vi "arm_sine.vi"(9 "Peak Amp":dbl=1e-05 format="%#_6e", 10 "Freq":dbl=71.34 format="%#_6e", 11 "Keithley":refnum<visa-resource-name>="GPIB1::22::INSTR") -> ()   [LabVIEW 2019]
uses:
  SineGlobals.vi
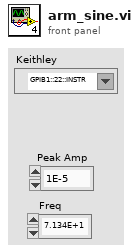
[diagram p1: front panel]
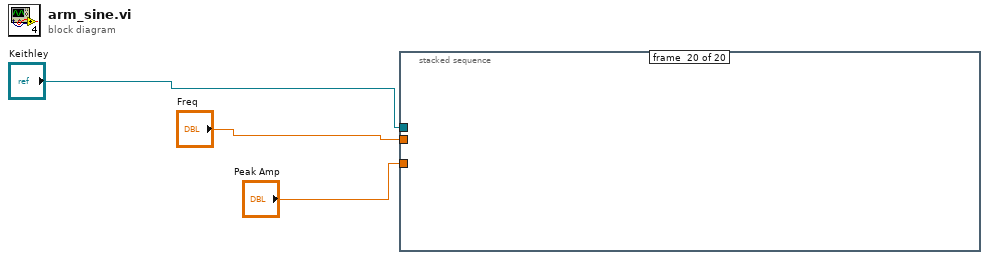
[diagram p0: block diagram]
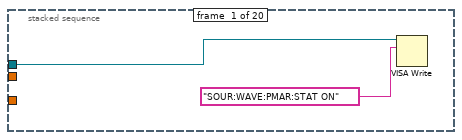
[diagram p2: hidden frame]
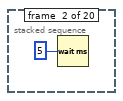
[diagram p3: hidden frame]
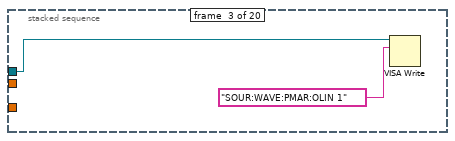
[diagram p4: hidden frame]
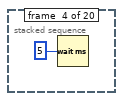
[diagram p5: hidden frame]
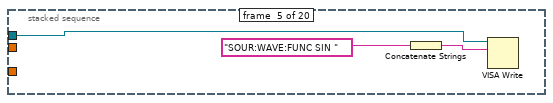
[diagram p6: hidden frame]
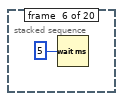
[diagram p7: hidden frame]
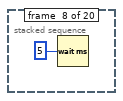
[diagram p9: hidden frame]
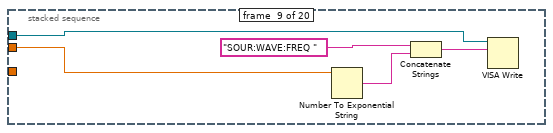
[diagram p10: hidden frame]
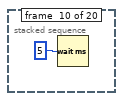
[diagram p11: hidden frame]
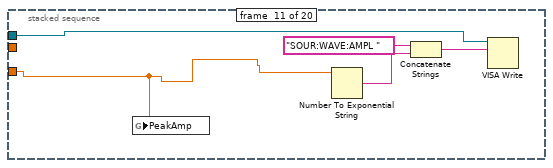
[diagram p12: hidden frame]
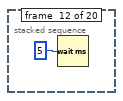
[diagram p13: hidden frame]
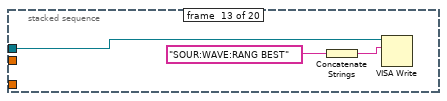
[diagram p14: hidden frame]
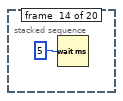
[diagram p15: hidden frame]
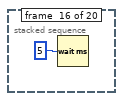
[diagram p17: hidden frame]
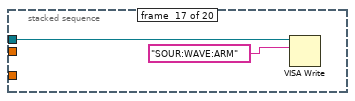
[diagram p18: hidden frame]
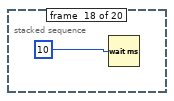
[diagram p19: hidden frame]
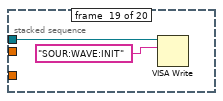
[diagram p20: hidden frame]
diagram:
  n1 = stacked-sequence {
    tunnel: "Freq" -> [_ _ _ _ _ _ _ _ w17 _ _ _ _ _ _ _ _ _ _ _]
    tunnel: "Keithley" -> [w4 _ w7 _ w10 _ _ _ w15 _ w22 _ w27 _ _ _ w32 _ w35 _]
    tunnel: "Peak Amp" -> [_ _ _ _ _ _ _ _ _ _ w21 _ _ _ _ _ _ _ _ _]
    frame #0 {
      n2 = VISA Write(VISA resource name=w4, write buffer="SOUR:WAVE:PMAR:STAT ON") -> ()  [unwired: 1 in, 3 out]
    }
    frame #1 {
      n3 = Wait (ms)(milliseconds to wait=5) -> ()  [unwired: 1 out]
    }
    frame #2 {
      n4 = VISA Write(VISA resource name=w7, write buffer="SOUR:WAVE:PMAR:OLIN 1") -> ()  [unwired: 1 in, 3 out]
    }
    frame #3 {
      n5 = Wait (ms)(milliseconds to wait=5) -> ()  [unwired: 1 out]
    }
    frame #4 {
      n6 = Concatenate Strings("SOUR:WAVE:FUNC SIN ") -> (w11:string)
      n7 = VISA Write(VISA resource name=w10, write buffer=w11) -> ()  [unwired: 1 in, 3 out]
    }
    frame #5 {
      n8 = Wait (ms)(milliseconds to wait=5) -> ()  [unwired: 1 out]
    }
    frame #6 {
    }
    frame #7 {
      n9 = Wait (ms)(milliseconds to wait=5) -> ()  [unwired: 1 out]
    }
    frame #8 {
      n10 = Number To Exponential String(number=w17) -> (E-format string=w18:string)  [unwired: 3 in]
      n11 = Concatenate Strings("SOUR:WAVE:FREQ ", w18) -> (w16:string)
      n12 = VISA Write(VISA resource name=w15, write buffer=w16) -> ()  [unwired: 1 in, 3 out]
    }
    frame #9 {
      n13 = Wait (ms)(milliseconds to wait=5) -> ()  [unwired: 1 out]
    }
    frame #10 {
      n14 = global write "SineGlobals.vi" "PeakAmp"(w21) -> ()
      n15 = Number To Exponential String(number=w21) -> (E-format string=w24:string)  [unwired: 3 in]
      n16 = Concatenate Strings("SOUR:WAVE:AMPL ", w24) -> (w23:string)
      n17 = VISA Write(VISA resource name=w22, write buffer=w23) -> ()  [unwired: 1 in, 3 out]
    }
    frame #11 {
      n18 = Wait (ms)(milliseconds to wait=5) -> ()  [unwired: 1 out]
    }
    frame #12 {
      n19 = Concatenate Strings("SOUR:WAVE:RANG BEST") -> (w28:string)
      n20 = VISA Write(VISA resource name=w27, write buffer=w28) -> ()  [unwired: 1 in, 3 out]
    }
    frame #13 {
      n21 = Wait (ms)(milliseconds to wait=5) -> ()  [unwired: 1 out]
    }
    frame #14 {
    }
    frame #15 {
      n22 = Wait (ms)(milliseconds to wait=5) -> ()  [unwired: 1 out]
    }
    frame #16 {
      n23 = VISA Write(VISA resource name=w32, write buffer="SOUR:WAVE:ARM") -> ()  [unwired: 1 in, 3 out]
    }
    frame #17 {
      n24 = Wait (ms)(milliseconds to wait=10) -> ()  [unwired: 1 out]
    }
    frame #18 {
      n25 = VISA Write(VISA resource name=w35, write buffer="SOUR:WAVE:INIT") -> ()  [unwired: 1 in, 3 out]
    }
    frame #19 {
    }
  }
